vi "ASCENDING AND DESCENDING USING ARRAYS.vi"() -> ()   [LabVIEW 2018]
panel:
  out "DESCENDING":dbl[](array[numeric])
  out "ASCENDING":dbl[](array[numeric])
  in  "Array":dbl[](array[numeric])
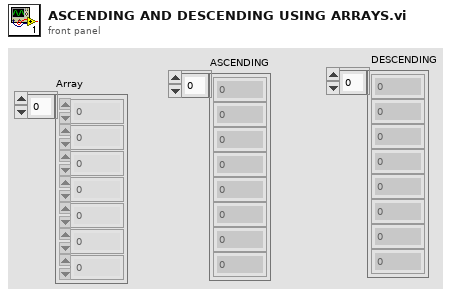
[diagram p1: front panel]
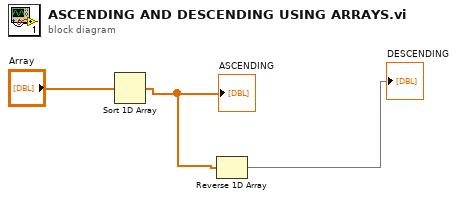
[diagram p0: block diagram]
diagram:
  n1 = Sort 1D Array(array="Array") -> (sorted array=w1:dbl[])
  "ASCENDING" <- w1
  n2 = Reverse 1D Array(array=w1) -> (reversed array=→"DESCENDING":dbl[])
